vi "Webservice Error Codes.vi"() -> (2 "webservice error descriptions":string[](array[string]), 3 "webservice error codes":i32[](array[numeric]))   [LabVIEW 2014, in "lvwd-components-start-utilities.lvlib"]
doc: "Used as one way of several to store error messages specific to the web application.\n\nReturns an array of error messages and corresponding error codes that can be used by General Error Handler."
uses:
  lvwd-components-start-utilities.lvlib
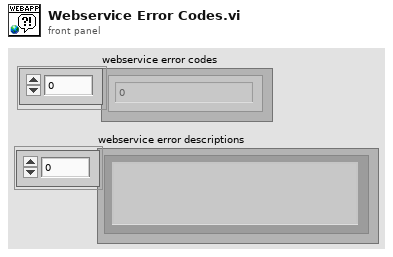
[diagram p1: front panel]
types:
  T1 = cluster{"error code":i32, "description":string}[]
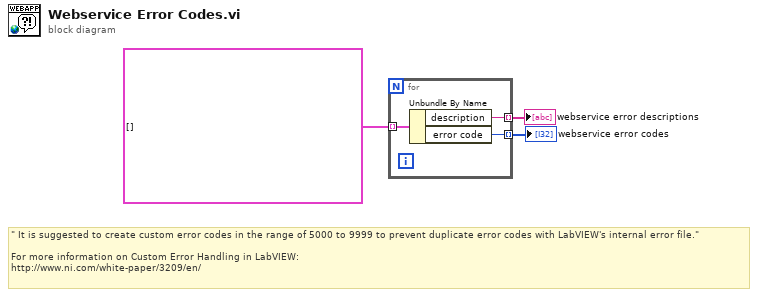
[diagram p0: block diagram]
diagram:
  # "\" It is suggested to create custom error codes in the range of 5000 to 9999 to prevent duplicate error codes with LabVIEW's internal error file.\"\n\nFor more information on Custom Error Handling in LabVIEW:\nhttp://www.ni.com/white-paper/3209/en/"
  n1 = for {
    tunnel: T1 [] ("Webservice Error Codes") -> [w6] mode=indexing
    tunnel: [w5] -> w2 mode=indexing
    tunnel: [w4] -> w1 mode=indexing
    n2 = Unbundle By Name(w6) -> ("description"=w5:string, "error code"=w4:i32)
  }
  "webservice error descriptions" <- w2
  "webservice error codes" <- w1
